vi "Config DSP402.vi"(5 "Wait?":bool, 6 "CCMD COB-Id":u32, 7 "Node ID":u8, 8 "CANopen":refnum<class "CANopen.lvclass">, 9 "DSP402 in":refnum<class "DSP402.lvclass">) -> (3 "DSP402 out":refnum<class "DSP402.lvclass">)   [LabVIEW 2024, in "canopen.lvlib" / "DSP402.lvclass"]
doc: "Configures the main parameters. It must be called before any other VI to prepare the communication parameters."
uses:
  DSP402.lvclass
  CANopen/CANopen.lvclass
  DriveState.ctl
  DriveMode.ctl
  DSP402.lvclass/DSP402.ctl
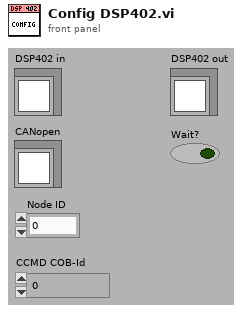
[diagram p1: front panel]
types:
  T1 = typedef "canopen.lvlib/DSP402.lvclass/DriveMode.ctl" = i8
  T2 = typedef "canopen.lvlib/DSP402.lvclass/DriveState.ctl" = enum16{"Start", "Not ready to switch on", "Switch on disabled", "Ready to switch on", "Switched on", "Operation enable", "Fault reaction active", "Fault", "Quick stop active"}
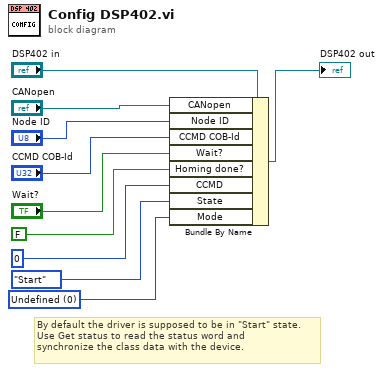
[diagram p0: block diagram]
diagram:
  w2 = T1 0 items=["Undefined"=0, "Profile Position Mode"=1, "Velocity Mode"=2, "Profile Velocity Mode"=3, "Torque Profile Mode"=4, "Homing Mode"=6, "Interpolated Position Mode"=7] ("Mode")
  # "By default the driver is supposed to be in \"Start\" state.\nUse Get status to read the status word and\nsynchronize the class data with the device."
  n1 = Bundle By Name(cluster="DSP402 in", "CANopen"="CANopen", "Node ID"="Node ID", "CCMD COB-Id"="CCMD COB-Id", "Wait?"="Wait?", "Homing done?"=FALSE, "CCMD"=u16 0, "State"=DriveState."Start", "Mode"=w2) -> (→"DSP402 out":refnum<class "DSP402.lvclass">)
